vi "Post_Dust_Event_Tick.vi"(7 "error in (no error)":errorcluster, 10 "Input Data":T1 {"Estimate Source" items=["Any Source."=-2, "No Shot"=-1, "Basic Labview Estimate"=0, "IDL Estimate From Andrew"=1, "IDL Estimate From Tobin"=2, "Old Metadata"=3]}) -> (0 "error out":errorcluster)   [LabVIEW 2013]
uses:
  <userlib>/Accelerator/User Interface/Controls/Dust_Event.ctl
  <userlib>/Accelerator/User Interface/Controls/Signal.ctl
  <userlib>/Accelerator/User Interface/Controls/Role ID.ctl
  <userlib>/Accelerator/User Interface/Controls/Hardware ID.ctl
  <userlib>/Accelerator/User Interface/Controls/Estimate_source.ctl
  <userlib>/_OpenG.lib/file/file.llb/File Exists - Scalar__ogtk.vi
panel:
  # "Dust Event"
  # "Signal"
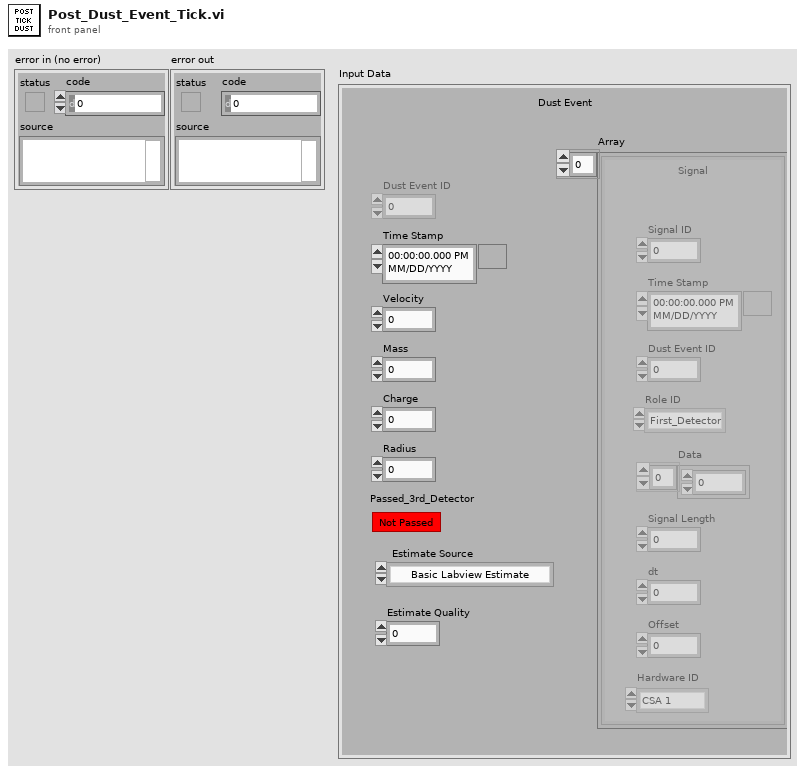
[diagram p1: front panel]
types:
  T1 = typedef "Dust_Event.ctl" = cluster{"Time Stamp":timestamp, "Velocity":sgl, "Mass":sgl, "Charge":sgl, "Radius":sgl, "Array":T2[], "Dust Event ID":i64, "Passed_3rd_Detector":bool, "Estimate Source":T5, "Estimate Quality":sgl}
  T2 = typedef "Signal.ctl" = cluster{"Signal ID":i64, "Time Stamp":timestamp, "Dust Event ID":i64, "Role ID":T3, "Data":sgl[], "Signal Length":i32, "dt":sgl, "Offset":dbl, "Hardware ID":T4}
  T3 = typedef "Role ID.ctl" = enum16{"First_Detector", "Second_Detector", "Third_Detector", "LeCroy_CH1", "LeCroy_CH2", "LeCroy_CH3", "LeCroy_CH4", "PSU", "DCS 1", "DCS 2"}
  T4 = typedef "Hardware ID.ctl" = enum16{"Unknown", "CSA 1", "CSA 2", "CSA 3", "CSA 4", "CSA 5", "CSA 6", "DCS 1", "DCS 2"}
  T5 = typedef "Estimate_source.ctl" = i8
  T6 = enum32{"Bad", "Idle", "Run top level", "Running"}
  T7 = typedef "Semaphore RefNum" = refnum<k1>
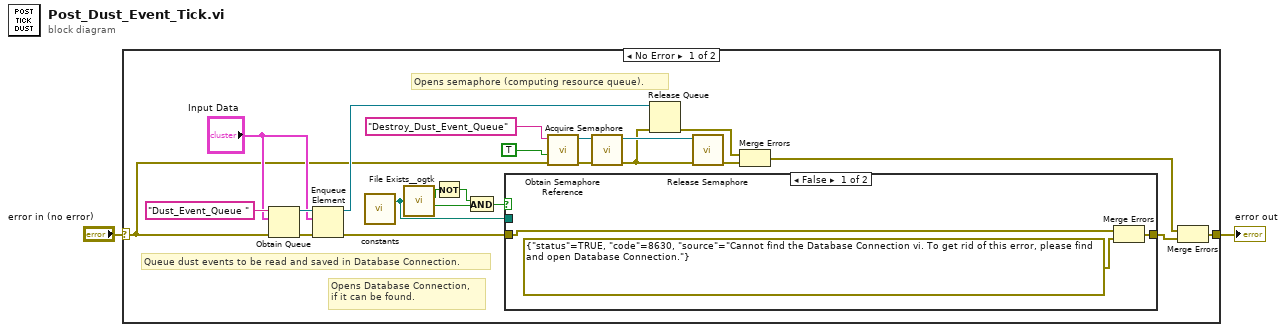
[diagram p0: block diagram]
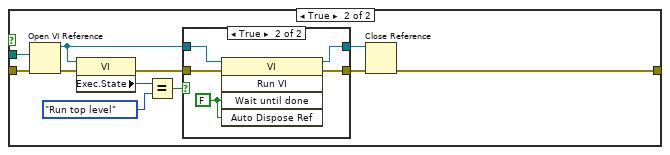
[diagram p2: hidden frame]
diagram:
  n1 = case shown="No Error" "error in (no error)" {
    selector: "error in (no error)" -> [w20 w47]
    tunnel: [w15 w47] -> w1
    frame No Error {
      # "Opens Database Connection,\nif it can be found."
      # "Queue dust events to be read and saved in Database Connection."
      # "Opens semaphore (computing resource queue)."
      n2 = Obtain Queue(name (unnamed)="Dust_Event_Queue ", element data type="Input Data", error in (no error)=w20) -> (queue out=w25:refnum<queue>, error out=w21:errorcluster)  [unwired: 2 in, 1 out]
      n3 = Enqueue Element(queue=w25, element="Input Data", error in (no error)=w21) -> (queue out=w23:refnum<queue>, error out=w3:errorcluster)  [unwired: 1 in, 1 out]
      n4 = call <userlib>:"constants.vi"() -> ("DB connection file path"=w4:path)  [unwired: 3 in, 2 out]
      n5 = call-poly <userlib>:"File Exists__ogtk.vi"("file path"=w4) -> ("is directory"=w7:bool, "exists"=w8:bool)  [unwired: 6 in]
      n6 = Not(x=w7) -> (.not. x?=w6:bool)
      n7 = And(x=w6, y=w8) -> (x .and. y?=w5:bool)
      n8 = case shown="False" w5 {
        tunnel: [w27 w31] -> w14
        tunnel: w3 -> [w28 w30]
        tunnel: w4 -> [_ w29]
        frame False {
          n9 = Merge Errors(w28, errorcluster {"status"=TRUE, "code"=8630, "source"="Cannot find the Database Connection vi. To get rid of this error, please find and open Database Connection."} ("error in")) -> (w27:errorcluster)
        }
        frame True {
          n10 = Open VI Reference(vi path=w29, error in (no error)=w30) -> (vi reference=w39:refnum<vi>, error out=w38:errorcluster)  [unwired: 4 in]
          n11 = property class="VI"(reference=w39, error in=w38) -> (error out=w37:errorcluster, "Exec.State"=w36:T6)  [unwired: 1 out]
          n12 = Equal?(x=w36, y=T6."Run top level" ("Execution:State")) -> (x = y?=w34:bool)
          n13 = case shown="True" w34 {
            tunnel: w39 -> [w40 w46]
            tunnel: w37 -> [w41 w45]
            tunnel: [w41 w44] -> w33
            tunnel: [w40 w43] -> w32
            frame False {
            }
            frame True {
              w42 = FALSE ("Wait Until Done")
              n14 = invoke class="VI" method="Run VI"(reference=w46, error in=w45, "Wait until done"=w42, "Auto Dispose Ref"=w42) -> (reference out=w43:refnum<vi>, error out=w44:errorcluster)  [unwired: 1 in, 3 out]
            }
          }
          n15 = Close Reference(reference=w32, error in (no error)=w33) -> (error out=w31:errorcluster)
        }
      }
      n16 = call <vilib>:"Obtain Semaphore Reference.vi"("error in (no error)"=w20, "create if not found (T)"=TRUE, "name (unnamed)"="Destroy_Dust_Event_Queue") -> ("error out"=w11:errorcluster, "semaphore"=w10:T7)  [unwired: 2 in, 1 out]
      n17 = call <vilib>:"Acquire Semaphore.vi"("error in (no error)"=w11, "semaphore"=w10) -> ("error out"=w17:errorcluster, "semaphore out"=w18:T7)  [unwired: 3 in, 1 out]
      n18 = Release Queue(queue=w23, error in (no error)=w17) -> (error out=w19:errorcluster)  [unwired: 1 in, 2 out]
      n19 = call <vilib>:"Release Semaphore.vi"("error in (no error)"=w17, "semaphore"=w18) -> ("error out"=w9:errorcluster)  [unwired: 4 in, 1 out]
      n20 = Merge Errors(w19, w9) -> (w16:errorcluster)
      n21 = Merge Errors(w16, w14) -> (w15:errorcluster)
    }
    frame Error {
    }
  }
  "error out" <- w1
